vi "WPI_IMU_IMUReset.vi"(6 "AHRS Reset In":dbl, 7 "Absolute Angle":dbl(slide) scale=-180.0..180.0, 8 "Reset":bool) -> (0 "AHRS Reset Out":dbl, 1 "Converted Output":dbl(slide) scale=-180.0..180.0)   [LabVIEW 2015, in "FRC ADI MXP IMU.lvlib"]
uses:
  FRC ADI MXP IMU.lvlib
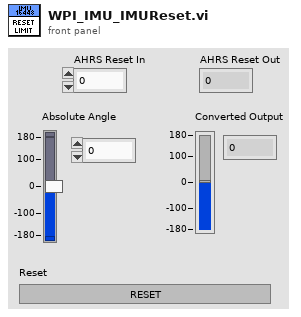
[diagram p1: front panel]
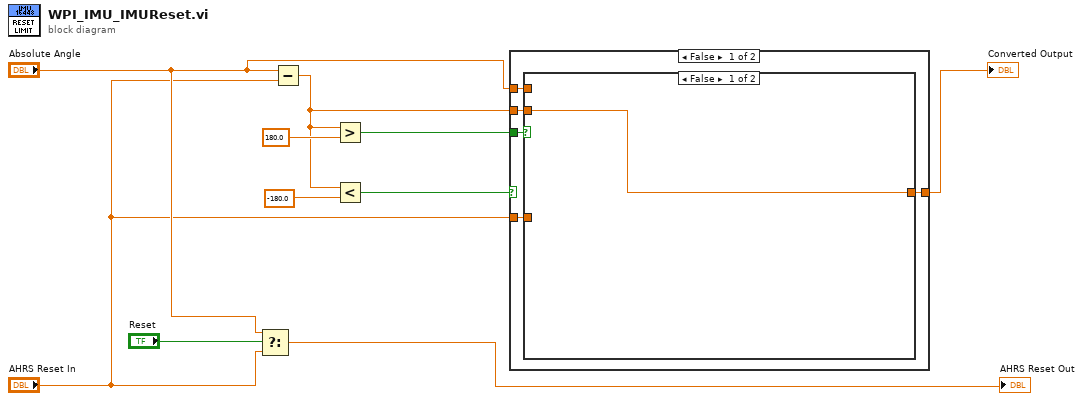
[diagram p0: block diagram]
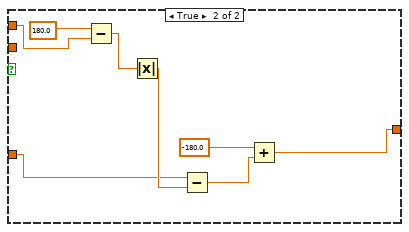
[diagram p2: hidden frame]
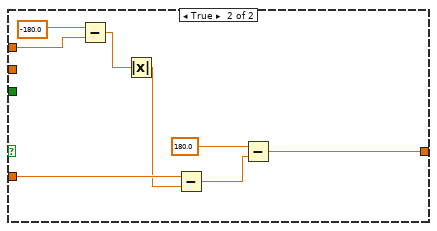
[diagram p3: hidden frame]
diagram:
  n1 = Select(t="Absolute Angle", s="Reset", f="AHRS Reset In") -> (s? t:f=→"AHRS Reset Out":dbl)
  n2 = Subtract(x="Absolute Angle", y="AHRS Reset In") -> (x-y=w5:dbl)
  n3 = Greater?(x=w5, y=180.0) -> (0:w6:bool)
  n4 = Less?(x=w5, y=-180.0) -> (x < y?=w8:bool)
  n5 = case shown="False" w8 {
    tunnel: "AHRS Reset In" -> [w14 w31]
    tunnel: "Absolute Angle" -> [w15 w29]
    tunnel: [w13 w25] -> w7
    tunnel: w6 -> [w12 _]
    tunnel: w5 -> [w11 _]
    frame False {
      n6 = case shown="False" w12 {
        tunnel: w15 -> [_ w18]
        tunnel: w14 -> [_ w19]
        tunnel: [w16 w17] -> w13
        tunnel: w11 -> [w16 _]
        frame False {
        }
        frame True {
          n7 = Subtract(x=180.0, y=w18) -> (x-y=w22:dbl)
          n8 = Absolute Value(x=w22) -> (abs(x)=w21:dbl)
          n9 = Subtract(x=w19, y=w21) -> (x-y=w20:dbl)
          n10 = Add(x=-180.0, y=w20) -> (x+y=w17:dbl)
        }
      }
    }
    frame True {
      n11 = Subtract(x=-180.0, y=w29) -> (x-y=w28:dbl)
      n12 = Absolute Value(x=w28) -> (abs(x)=w27:dbl)
      n13 = Subtract(x=w31, y=w27) -> (x-y=w26:dbl)
      n14 = Subtract(x=180.0, y=w26) -> (x-y=w25:dbl)
    }
  }
  "Converted Output" <- w7
